vi "CNC Main.vi"() -> ()   [LabVIEW 2014]
uses:
  Typedefs/DXF Choices.ctl
  Typedefs/Demo States.ctl
  Typedefs/Motion Parameters.ctl
  <vilib>/Motion/Express/_s/nimc.fb.straightLineMove.blendMode.ctl
  Typedefs/GCode Choices.ctl
  Typedefs/GCode Scale Options.ctl
  Typedefs/DXF Scale Options.ctl
  Typedefs/Message.ctl
  Typedefs/Demo Actions.ctl
  GCode Parser/GCode Command Cluster.ctl
  <vilib>/Motion/Express/_s/nimc.ex.read.readTrajectoryData.coordinate.vi
  <vilib>/Motion/Express/_s/nimc.ex.read.readTrajectoryData.axis.vi
  <vilib>/Motion/Express/_s/nimc.ex.straightLineMove.startStraightLineMove.coordinate.modeRelative.0.vi
  <vilib>/Motion/Express/_s/nimc.ex.resetPosition.resetPosition.coordinate.vi
  <vilib>/Motion/Express/_s/nimc.ex.straightLineMove.startStraightLineMove.coordinate.modeAbsolute.0.vi
  <vilib>/Motion/Express/_s/nimc.ex.read.readExecutionData.coordinate.vi
  <vilib>/Motion/Express/_s/nimc.ex.stopMove.stop.coordinate.modeDecelerate.vi
  <vilib>/Motion/BlockNode/FB.NIMotion.xnode
  Functional_Global/Typedef_FPGA_Interface_Action.ctl
  <vilib>/ptbypt/NI_PtbyPt.lvlib
panel:
  in  "GCode Choices":T1=enum."Statue"
  in  "DXF Choices 2":enum16{"NI Logo", "Mermaid", "Hummingbird"}(ring)
  in  "DXF Debug":T2={"Pos Scale"=30.0, "X Offset"=-350.0, "Y Offset"=-350.0}
  in  "GCODE Debug":T3={"Pos Scale"=8.0, "Vel Scale"=8.0, "G0 Velocity"=800.0, "X Offset"=0.0, "Y Offset"=0.0, "Z Offset"=0.0}
  in  "OK Button":bool
  in  "OK Button 2":bool
  in  "OK Button 3":bool
  in  "OK Button 4":bool
  in  "OK Button 5":bool
  in  "OK Button 6":bool
  in  "Pause":bool
  out "Axis Positions":T4(graph)
  in  "Disable Graph Update":bool
  in  "Clear XY Graph":bool
  out "# in queue":i32
  out "pos.[] out":dbl[](array[numeric]) format="%#.2f"
  out "Demo States":T5
  in  "Global Stop":bool=TRUE
  out "GCODE":i32(listbox)=-1
  in  "Tab":enum32{"DXF", "GCODE", "Setup", "Debug"}(tab)
  in  "DXF Scale Options":T2[](array[typedef])=[{"Pos Scale"=250.0, "X Offset"=-1025.0, "Y Offset"=-1500.0}, {"Pos Scale"=75.0, "X Offset"=-180.0, "Y Offset"=-300.0}, {"Pos Scale"=30.0, "X Offset"=-350.0, "Y Offset"=-350.0}]
  in  "DXF Options":T6={"Pen Up Z"=50.0, "Pen Down Z"=-10.0, "Speed"=1500.0, "Z Move Speed"=300.0}
  in  "Start DXF":bool
  in  "DXF Choices":T7 items=["NI Logo", "Mermaid", "Hummingbird", ""]
  in  "GCODE Scale Options":T3[](array[typedef])=[{"Pos Scale"=20.0, "Vel Scale"=20.0, "G0 Velocity"=800.0, "X Offset"=0.0, "Y Offset"=0.0, "Z Offset"=0.0}, {"Pos Scale"=2.0, "Vel Scale"=1.0, "G0 Velocity"=800.0, "X Offset"=-225.0, "Y Offset"=-225.0, "Z Offset"=0.0}, {"Pos Scale"=7.0, "Vel Scale"=7.0, "G0 Velocity"=800.0, "X Offset"=0.0, "Y Offset"=0.0, "Z Offset"=0.0}]
  in  "Start GCode":bool
  in  "GCODE Choices":T7 items=["Letter S", "Scorpion", "Statue", "", ""]
  in  "Set Home Point":bool
  in  "Reset Position":bool
  out "Error":errorcluster
  in  "Update Rate (ms)":u32=20
  in  "Buffer size":i32=2000
  in  "Cell Font:Size":u32=24
  in  "Display Row":i32=6
  out "stored home position":dbl[](array[numeric])
  in  "Quit":bool
  in  "Reset to":dbl[](array[numeric])=[0.0, 0.0, 0.0, 0.0]
  in  "Axis Resources":refnum<k21>[](array[refnum])=["Axis 1", "Axis 2", "Axis 3", "Axis 4"]
  out "Request Parameters":T8={"timeout"=-1.0, "acceleration"=8000.0, "deceleration"=8000.0, "accel. jerk"=80000.0, "decel. jerk"=80000.0, "blend mode"=10551334, "blend delay"=-1.0, "smoothing"=0.5, "last blend"=FALSE} {"blend mode" items=["At Profile Complete"=10551335, "At Deceleration"=10551334, "After Delay"=10551336]}
  in  "Acc Multiplier":dbl=10.0 format="%#_13g"
  in  "Jerk Multiplier":dbl=100.0 format="%#_13g"
  in  "Coordinate Space":refnum<k21>="Coordinate Space 1"
  out "F":dbl=800.0
  in  "Move (debug)":bool
  in  "debug velocity":dbl=750.0
  in  "debug pos":dbl[](array[numeric])=[0.0, 0.0, -200.0, 0.0]
  in  "VEL %":dbl(slide)=1.0 min=0.01 max=1000.0 scale=0.01..100.0
  in  "Find Home":bool
  out "XY Graph":cluster{"X Array":dbl[], "Y Array":dbl[]}(graph)
  in  "Stop":bool
  out "Axis Velocities":T10(graph)
  # "scorpion:\n\nPOs: 2.5\nVel: 1\n\nAcc/Dec: 50000\nJerk: 500000\n\nG0: 800"
  # "X"
  # "Y"
  # "Z"
  # "Status:"
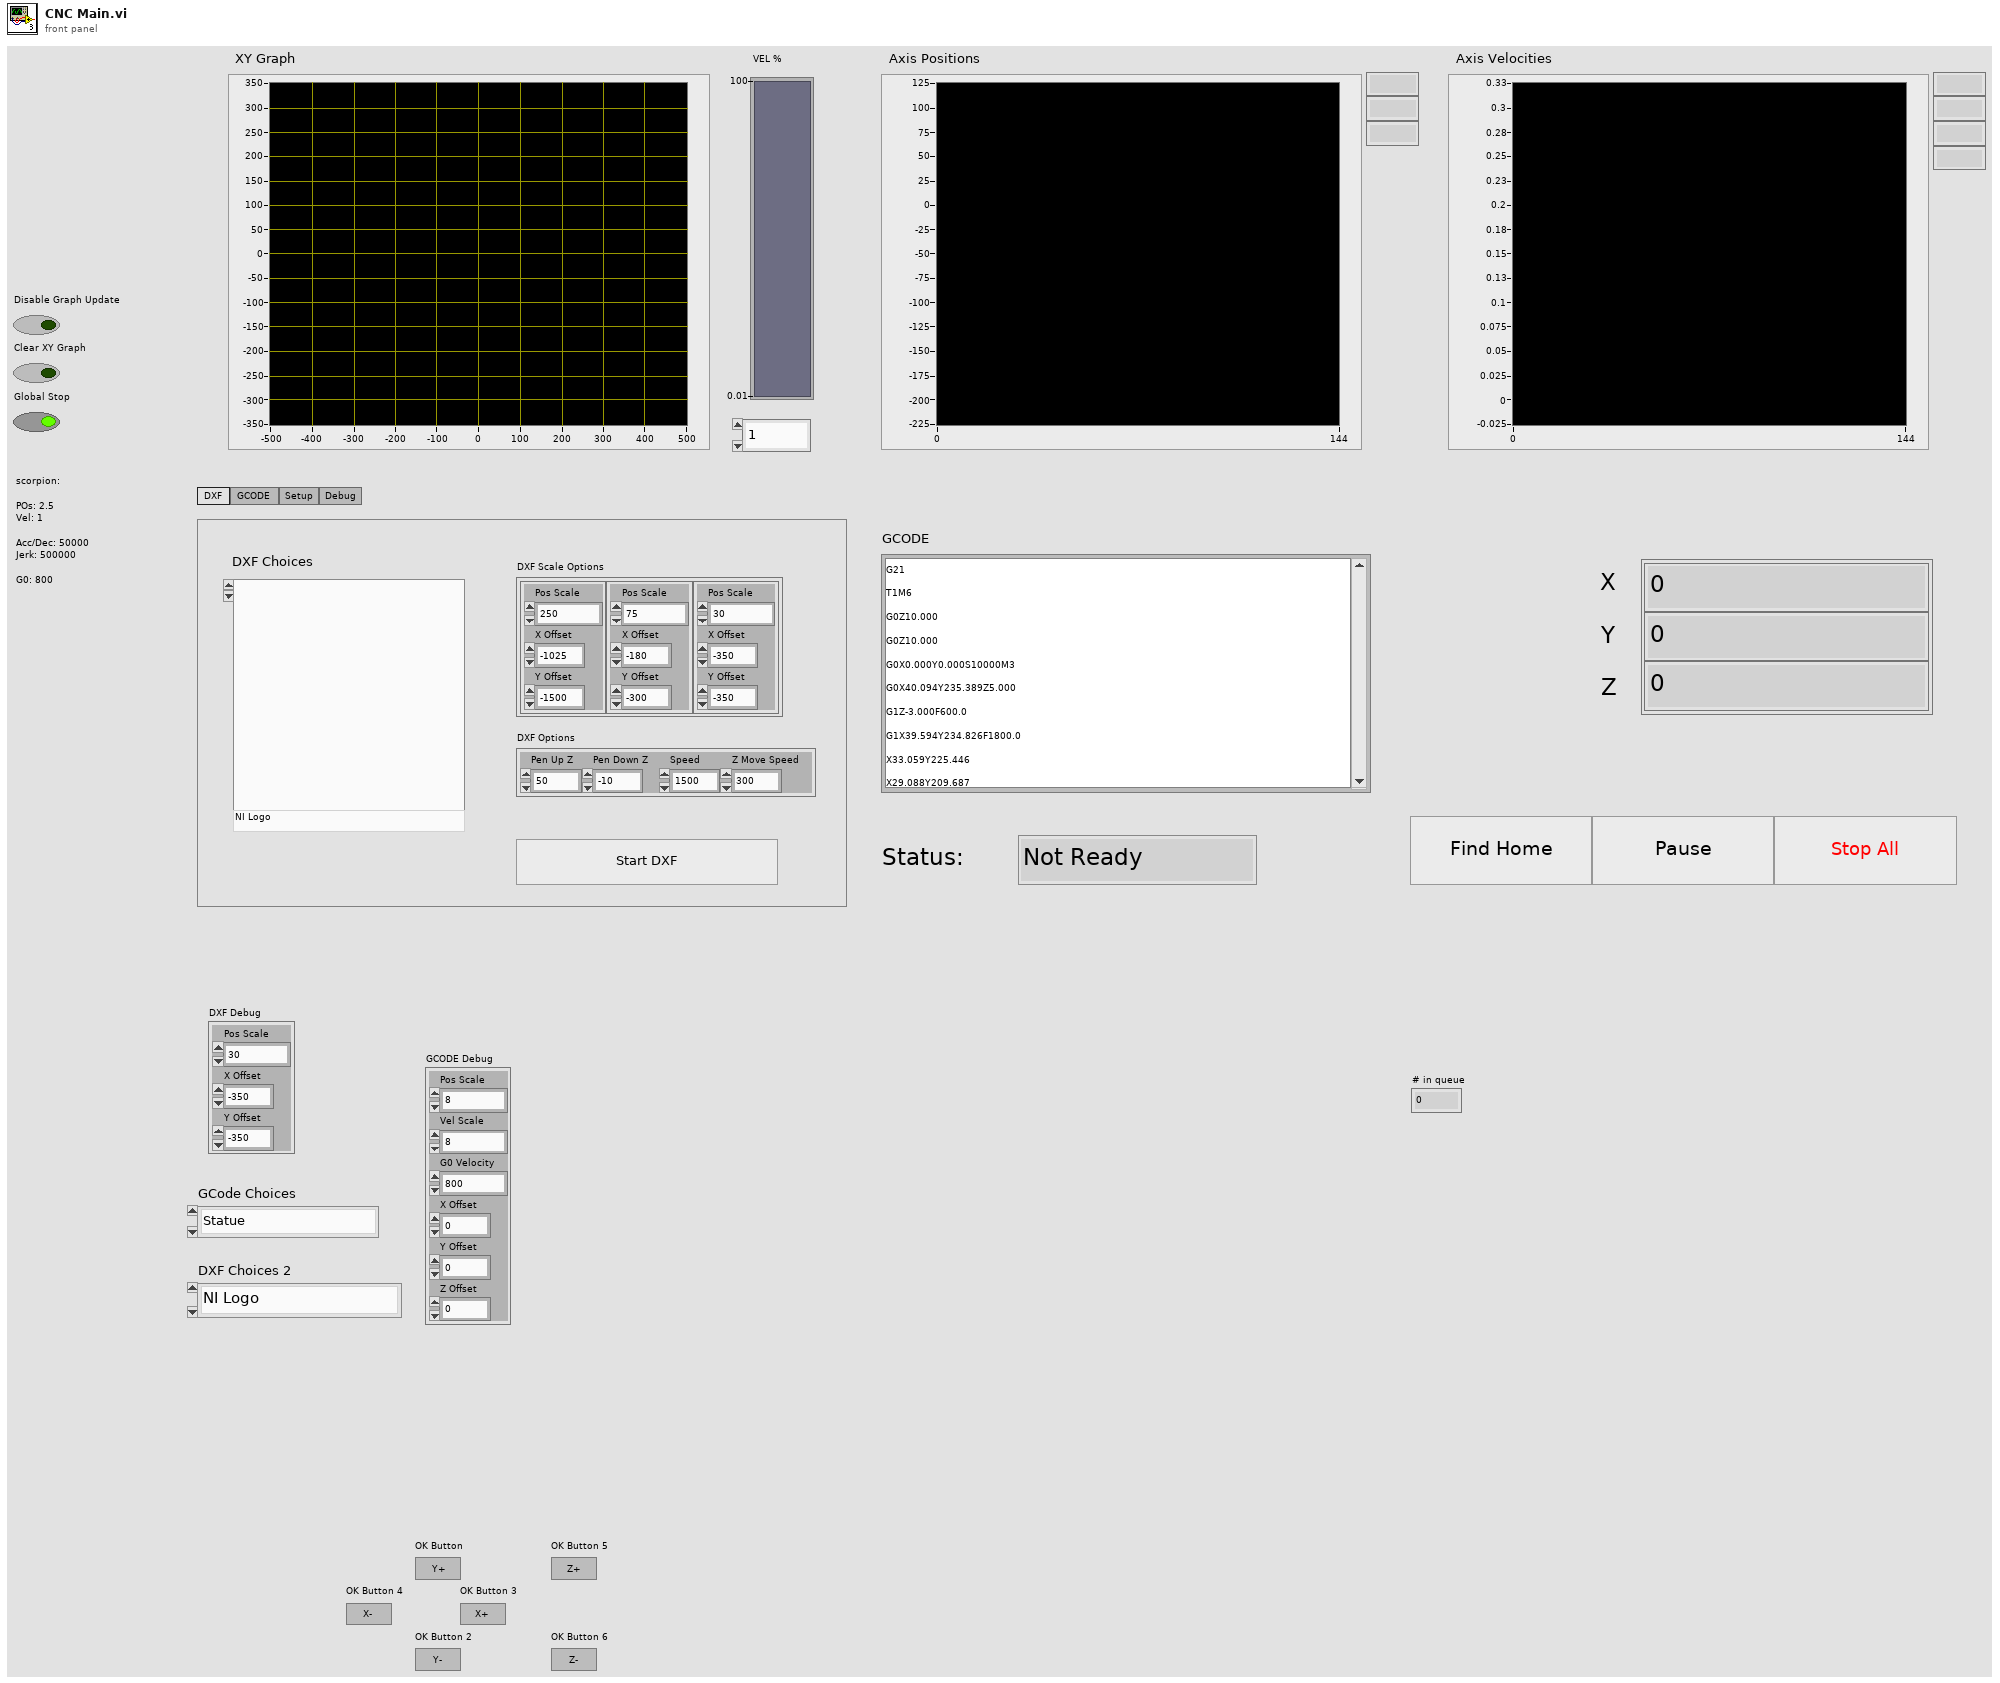
[diagram p1: front panel]
types:
  T1 = typedef "GCode Choices.ctl" = enum16{"S", "Scorpion", "Statue"}
  T2 = typedef "DXF Scale Options.ctl" = cluster{"Pos Scale":dbl, "X Offset":dbl, "Y Offset":dbl}
  T3 = typedef "GCode Scale Options.ctl" = cluster{"Pos Scale":dbl, "Vel Scale":dbl, "G0 Velocity":dbl, "X Offset":dbl, "Y Offset":dbl, "Z Offset":dbl}
  T4 = cluster{"commanded pos.[] out[0]":dbl, "commanded pos.[] out[1]":dbl, "commanded pos.[] out[2]":dbl}
  T5 = typedef "Demo States.ctl" = enum16{"Not Ready", "Ready (Idle)", "Running", "Paused"}
  T6 = cluster{"Pen Up Z":dbl, "Pen Down Z":dbl, "Speed":dbl, "Z Move Speed":dbl}
  T7 = typedef "DXF Choices.ctl" = u16
  T8 = typedef "Motion Parameters.ctl" = cluster{"timeout":dbl, "acceleration":dbl, "deceleration":dbl, "accel. jerk":dbl, "decel. jerk":dbl, "blend mode":T9, "blend delay":dbl, "smoothing":dbl, "last blend":bool}
  T9 = typedef "nimc.fb.straightLineMove.blendMode.ctl" = i32
  T10 = cluster{"[0]":dbl, "[1]":dbl, "[2]":dbl, "[3]":dbl}
  T11 = typedef "GCode Command Cluster.ctl" = cluster{"N":dbl, "GCODE":string, "X":dbl, "Y":dbl, "Z":dbl, "E":dbl, "I":dbl, "J":dbl, "S":dbl, "F":dbl, "Text":string, "G0 Vel":dbl}
  T12 = typedef "Message.ctl" = cluster{"Demo Actions":T13, "Data":variant}
  T13 = typedef "Demo Actions.ctl" = enum16{"Default (Null)", "Move (debug)", "Reset Position", "Find Home and Move to Zero", "Set Home Point", "Start", "Stop", "Pause", "Unpause"}
  T14 = typedef "Typedef_FPGA_Interface_Action.ctl" = enum16{"Initialize FPGA", "Get FPGA Reference", "Close FPGA"}
  T15 = enum8{"Enabled", "Disabled", "Disabled and Grayed Out"}
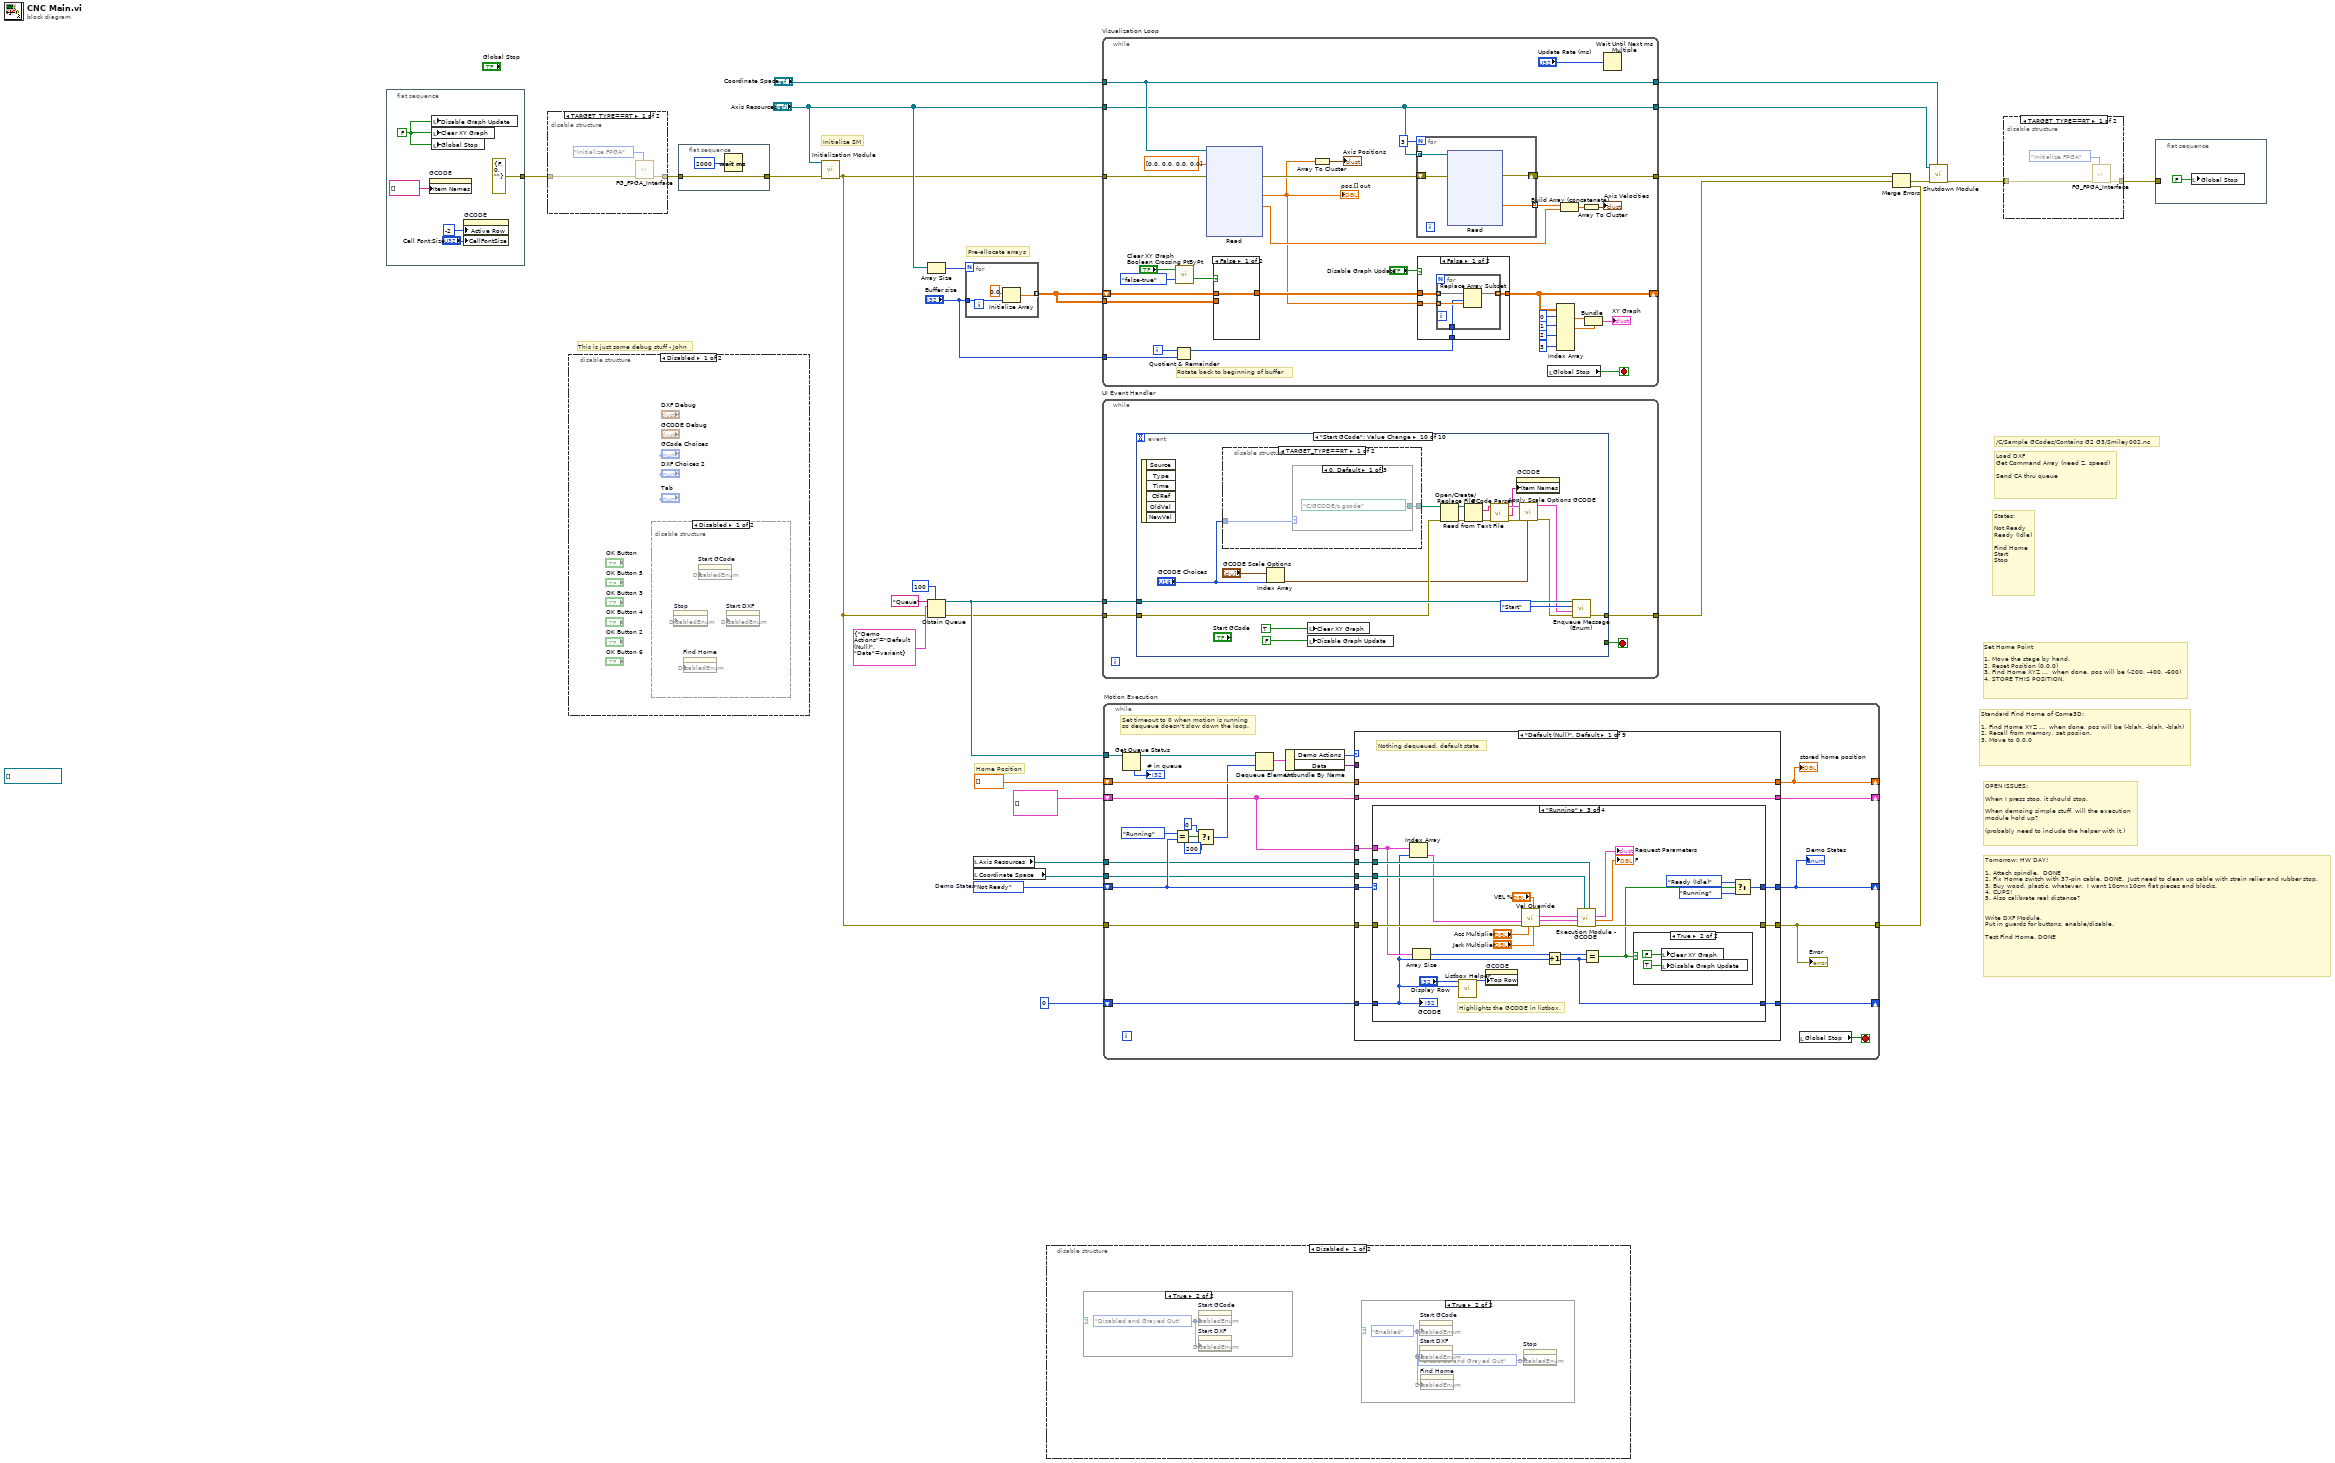
[diagram p0: block diagram]
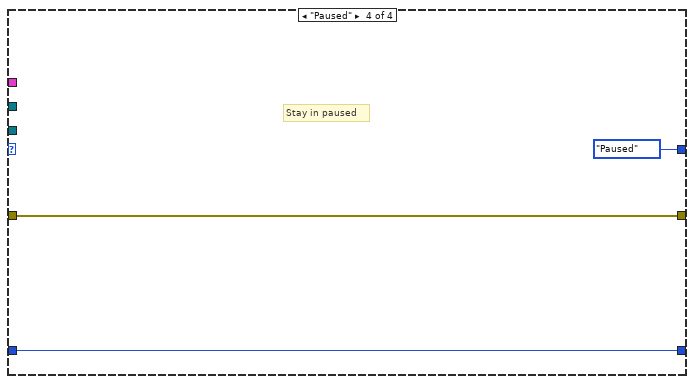
[diagram p12: hidden frame]
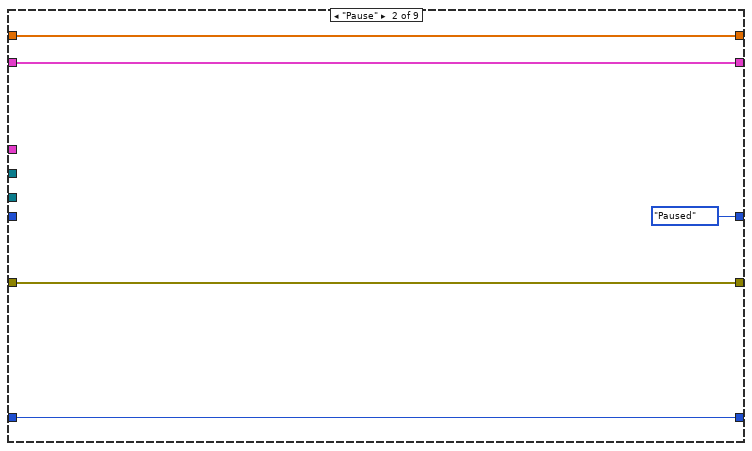
[diagram p13: hidden frame]
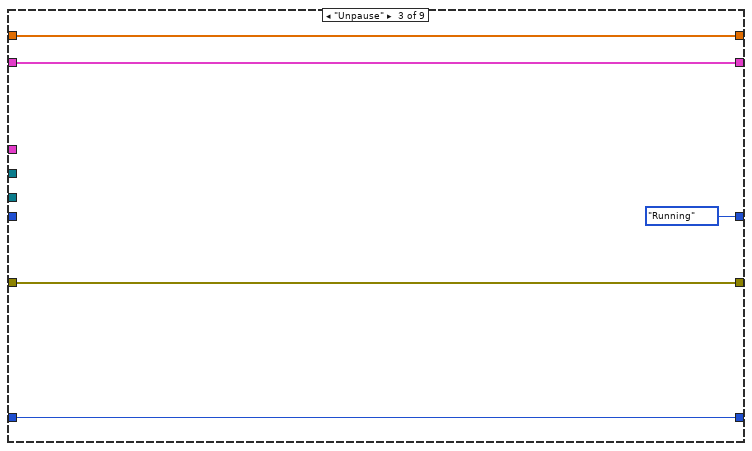
[diagram p14: hidden frame]
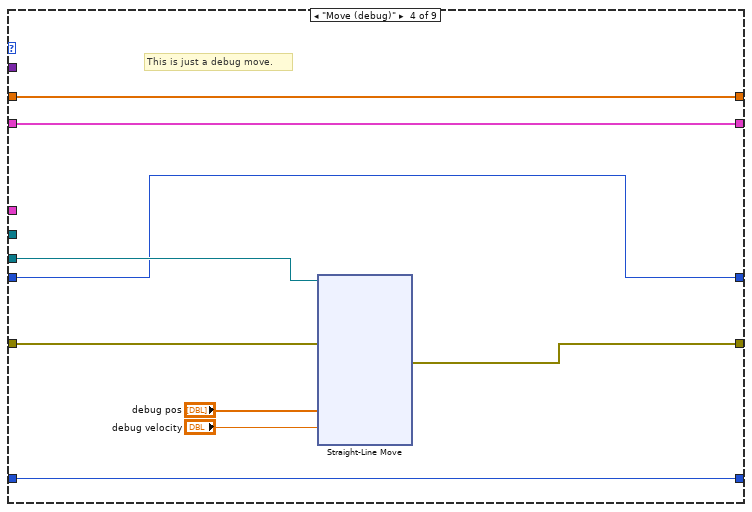
[diagram p15: hidden frame]
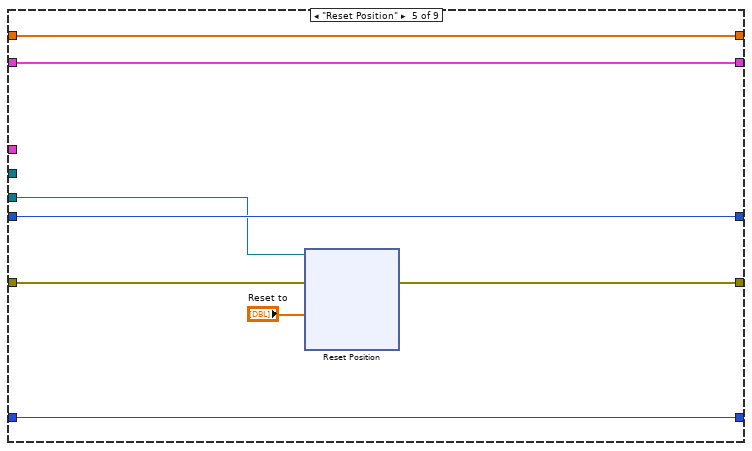
[diagram p16: hidden frame]
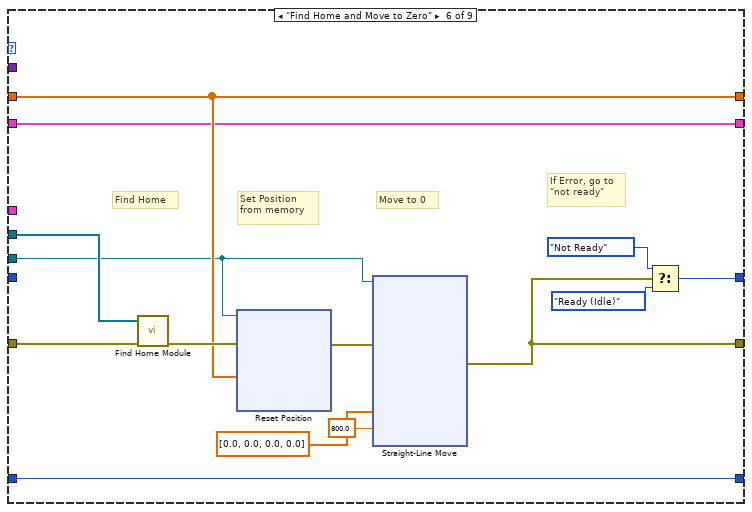
[diagram p17: hidden frame]
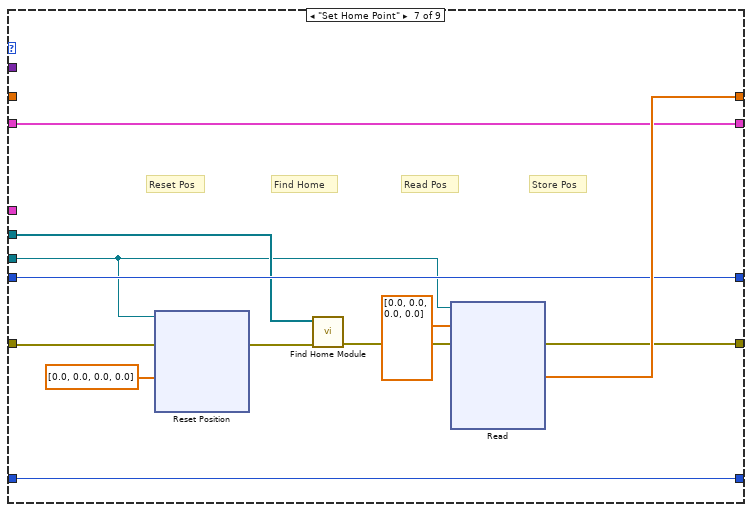
[diagram p18: hidden frame]
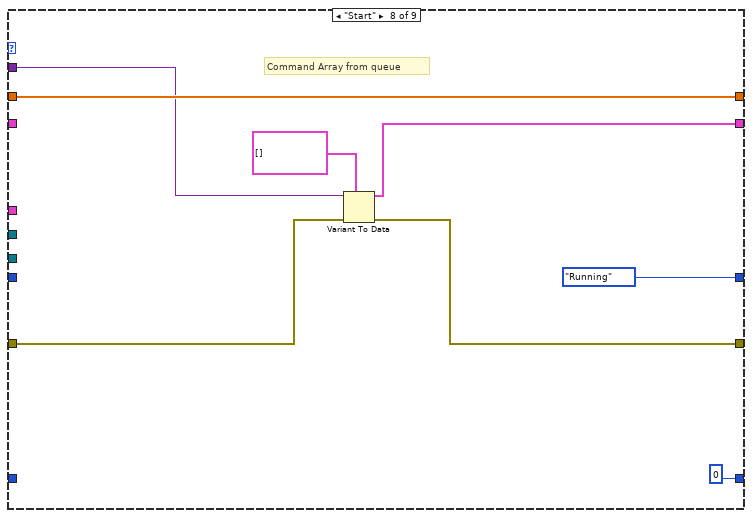
[diagram p19: hidden frame]
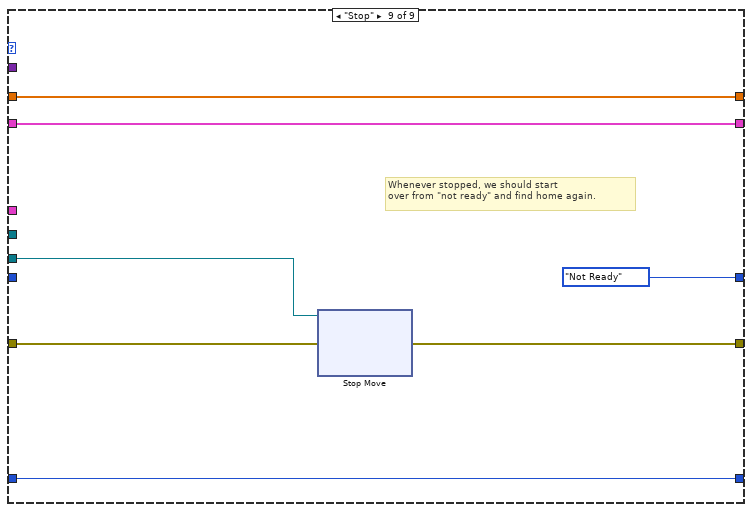
[diagram p20: hidden frame]
diagram:
  w4 = Demo_States."Not Ready"  # Demo States
  (unwired) refnum<k21>[] []
  # "This is just some debug stuff - John"
  # "Tomorrow: HW DAY!\n\n1. Attach spindle.  DONE\n2. Fix Home switch with 37-pin cable. DONE.  Just need to clean up cable with strain relier and rubber stop.\n3. Buy wood, plastic, whatever.  I want 10cmx10cm flat pieces and blocks.\n4. CLIPS!\n5. Also calibrate real distance?\n\n\nWrite DXF Module.\nPut in guards for buttons, enable/disable.\n\nTest Find Home. DONE"
  # "OPEN ISSUES:\n\nWhen I press stop, it should stop.\n\nWhen demoing simple stuff, will the execution \nmodule hold up?\n\n(probably need to include the helper with it.)"
  # "/C/Sample GCodes/Contains G2 G3/Smiley002.nc"
  # "Home Position"
  # "Pre-allocate arrays"
  # "Standard Find Home of Come3D:\n\n1. Find Home XYZ ...  when done, pos will be (-blah, -blah, -blah)\n2. Recall from memory, set posiion.\n3. Move to 0,0,0"
  # "Set Home Point\n\n1. Move the stage by hand.\n2. Reset Position (0,0,0)\n3. Find Home XYZ ...  when done, pos will be (-200, -400, -600)\n4. STORE THIS POSITION."
  # "Load DXF\nGet Command Array (need Z, speed)\n\nSend CA thru queue"
  # "States:\n\nNot Ready\nReady (Idle)\n\nFind Home\nStart\nStop"
  # "Initialize SM"
  n1 = flat-sequence {
    tunnel: [errorcluster {"status"=FALSE, "code"=0, "source"=""} ("error in")] -> w20
    frame #0 {
      w30 = FALSE ("Global Stop")
      n2 = property on="GCODE" class="LstBox (strict)"("Item Names"=string[] []) -> ()  [unwired: 2 in, 2 out]
      n3 = local write "Disable Graph Update"(w30) -> ()
      n4 = local write "Clear XY Graph"(w30) -> ()
      n5 = local write "Global Stop"(w30) -> ()
      n6 = property on="GCODE" class="LstBox (strict)"("Active Row"=-2 ("Active Row:Active Row Number"), "CellFontSize"="Cell Font:Size") -> ()  [unwired: 2 in, 2 out]
    }
  }
  n7 = disable-structure shown="TARGET_TYPE==RT" {
    disable-tunnel: [w35 w37] -> w28
    disable-tunnel: w20 -> [w34 w37]
    frame condition #0 {
      n8 = call "FG_FPGA_Interface.vi"("Action"=Typedef_FPGA_Interface_Action."Initialize FPGA", "error in"=w34) -> ("error out"=w35:errorcluster)  [unwired: 8 in, 1 out]
    }
    frame condition #1 (active) {
    }
  }
  n9 = disable-structure shown="Disabled" {
    frame Disabled {
      n10 = disable-structure shown="Disabled" {
        frame Disabled {
          n11 = property on="Stop" class="Bool" props=["DisabledEnum"]() -> ()  [unwired: 3 in, 2 out]
          n12 = property on="Find Home" class="Bool" props=["DisabledEnum"]() -> ()  [unwired: 3 in, 2 out]
          n13 = property on="Start GCode" class="Bool" props=["DisabledEnum"]() -> ()  [unwired: 3 in, 2 out]
          n14 = property on="Start DXF" class="Bool" props=["DisabledEnum"]() -> ()  [unwired: 3 in, 2 out]
        }
        frame Enabled {
        }
      }
    }
    frame Enabled {
    }
  }
  n15 = flat-sequence {
    tunnel: w28 -> [w38]
    tunnel: [w38] -> w25
    frame #0 {
      n16 = Wait (ms)(milliseconds to wait=u32 2000) -> ()  [unwired: 1 out]
    }
  }
  n17 = call "Initialization Module.vi"("error in (no error)"=w25, "Axis Resources In"="Axis Resources") -> ("error out"=w8:errorcluster)  [unwired: 8 in, 1 out]
  n18 = Array Size(array="Axis Resources") -> (size(s)=w27:i32)
  n19 = Obtain Queue(max queue size (-1, unlimited)=100, name (unnamed)="Queue", element data type=T12 {"Demo Actions"=enum."Default (Null)", "Data"=variant}, error in (no error)=w8) -> (queue out=w15:refnum<queue>, error out=w14:errorcluster)  [unwired: 1 in, 1 out]
  n20 = for {
    N: w27 -> [_]
    tunnel: [w41] -> w9 mode=indexing
    tunnel: "Buffer size" -> [w40]
    n21 = Initialize Array(0.0 ("element"), w40) -> (w41:dbl[])
  }
  n22 = local read "Axis Resources"() -> (w6:refnum<k21>[])
  n23 = local read "Coordinate Space"() -> (w5:refnum<k21>)
  n24 = disable-structure shown="Disabled" {
    frame Disabled {
      n25 = case shown="True" {
        selector: _ -> [_ _]
        frame False {
        }
        frame True {
          w43 = T15."Disabled and Grayed Out" ("Disabled")
          n26 = property on="Start GCode" class="Bool"("DisabledEnum"=w43) -> ()  [unwired: 2 in, 2 out]
          n27 = property on="Start DXF" class="Bool"("DisabledEnum"=w43) -> ()  [unwired: 2 in, 2 out]
        }
      }
      n28 = case shown="True" {
        selector: _ -> [_ _]
        frame False {
        }
        frame True {
          w45 = T15."Enabled" ("Disabled")
          n29 = property on="Start GCode" class="Bool"("DisabledEnum"=w45) -> ()  [unwired: 2 in, 2 out]
          n30 = property on="Start DXF" class="Bool"("DisabledEnum"=w45) -> ()  [unwired: 2 in, 2 out]
          n31 = property on="Find Home" class="Bool"("DisabledEnum"=w45) -> ()  [unwired: 2 in, 2 out]
          n32 = property on="Stop" class="Bool"("DisabledEnum"=T15."Disabled and Grayed Out" ("Disabled")) -> ()  [unwired: 2 in, 2 out]
        }
      }
    }
    frame Enabled {
    }
  }
  n33 = while "Visualization Loop" {
    tunnel: "Buffer size" -> [w78]
    tunnel: "Axis Resources" -> [w50]
    shift-right: [w59] -> _
    shift-left: w9 -> [w58]
    tunnel: "Coordinate Space" -> [w65]
    tunnel: [w50] -> w23
    tunnel: [w65] -> w24
    tunnel: w9 -> [w57]
    tunnel: w8 -> [w76]
    tunnel: [w74] -> w19
    i -> [w77]
    stop <- w62 stop-if-true
    # "Rotate back to beginning of buffer"
    n34 = Quotient & Remainder(x=w77, y=w78) -> (x-y*floor(x/y)=w73:i32)  [unwired: 1 out]
    n35 = call <vilib>:"Boolean Crossing PtByPt.vi"("direction"=enum16{"either", "false-true", "true-false"}."false-true", "input"="Clear XY Graph") -> ("crossing"=w54:bool)  [unwired: 1 in]
    n36 = xnode ("Read")("resource"=w65, "commanded pos.[]"=dbl[] [0.0, 0.0, 0.0, 0.0], "error in"=w76) -> ("commanded pos.[] out"=w46:dbl[], "commanded vel."=w49:dbl, "error out"=w75:errorcluster)  [unwired: 3 out]
    "pos.[] out" <- w46
    n37 = case shown="False" w54 {
      tunnel: w58 -> [w88 _]
      tunnel: w57 -> [_ w89]
      tunnel: [w88 w89] -> w56
      frame False {
      }
      frame True {
      }
    }
    n38 = Array To Cluster(array=w46) -> (cluster=→"Axis Positions":T4)
    n39 = for {
      N: 3 -> [_]
      tunnel: w50 -> [w102] mode=indexing
      tunnel: [w99] -> w61 mode=indexing
      shift-right: [w100] -> w74
      shift-left: w75 -> [w101]
      n40 = xnode ("Read")("resource"=w102, "error in"=w101) -> ("commanded vel."=w99:dbl, "error out"=w100:errorcluster)  [unwired: 3 out]
    }
    n41 = case shown="False" "Disable Graph Update" {
      tunnel: w73 -> [w82 _]
      tunnel: w46 -> [w81 _]
      tunnel: [w80 w87] -> w59
      tunnel: w56 -> [w79 w87]
      frame False {
        n42 = for {
          tunnel: w79 -> [w86] mode=indexing
          tunnel: w81 -> [w85] mode=indexing
          tunnel: w82 -> [w84]
          tunnel: [w83] -> w80 mode=indexing
          n43 = Replace Array Subset(array=w86, new element=w85, index=w84) -> (w83:dbl[])
        }
      }
      frame True {
      }
    }
    n44 = local read "Global Stop"() -> (w62:bool)
    n45 = Index Array(array=w59, index (row) #1=0 ("index (row)"), index (row) #2=1 ("index (row)"), index (row) #3=2 ("index (row)"), index (row) #4=3 ("index (row)")) -> (element #1=w68:dbl[], element #2=w69:dbl[])  [unwired: 4 in, 2 out]
    n46 = Build Array (concatenate)(w61, w49) -> (w60:dbl[])
    n47 = Array To Cluster(array=w60) -> (cluster=→"Axis Velocities":T10)
    n48 = Bundle(w68, w69) -> (→"XY Graph":cluster{dbl[], dbl[]})  [unwired: 1 in]
    n49 = Wait Until Next ms Multiple(millisecond multiple="Update Rate (ms)") -> ()  [unwired: 1 out]
  }
  n50 = while "UI Event Handler" {
    tunnel: w15 -> [w113]
    tunnel: w14 -> [w112]
    tunnel: [w111] -> w17
    stop <- w110 stop-if-true
    n51 = event shown="[9] \"Start GCode\": Value Change" {
      selector: _ -> [_ _ _ _ _ _ _ _ _ _]
      dyn-events: _ -> [_ _ _ _ _ _ _ _ _ _]
      timeout: _ -> [_ _ _ _ _ _ _ _ _ _]
      tunnel: w113 -> [_ w118 w122 w128 w135 w139 _ w146 w166 w203]
      tunnel: w112 -> [w114 w117 w121 w127 w134 w138 w142 w145 w162 w197]
      tunnel: [w114 w116 w120 w126 w133 w137 w142 w144 w165 w202] -> w111
      tunnel: [_ _ _ _ _ _ TRUE _ _ _] -> w110
      event Timeout {
        n52 = event-data() -> ()  [unwired: 1 in, 3 out]
      }
      event "Find Home": Value Change {
        n53 = event-data() -> ()  [unwired: 1 in, 6 out]
        n54 = call "Enqueue Message (Enum).vi"("error in (no error)"=w117, "Demo Actions"=Demo_Actions."Find Home and Move to Zero", "queue in"=w118) -> ("error out"=w116:errorcluster)  [unwired: 7 in, 1 out]
      }
      event "Set Home Point": Value Change {
        n55 = event-data() -> ()  [unwired: 1 in, 6 out]
        n56 = call "Enqueue Message (Enum).vi"("error in (no error)"=w121, "Demo Actions"=Demo_Actions."Set Home Point", "queue in"=w122) -> ("error out"=w120:errorcluster)  [unwired: 7 in, 1 out]
      }
      event "Stop": Value Change {
        n57 = event-data() -> ()  [unwired: 1 in, 6 out]
        n58 = call "Enqueue Message (Enum).vi"("error in (no error)"=w127, "Demo Actions"=Demo_Actions."Stop", "queue in"=w128) -> ("error out"=w126:errorcluster)  [unwired: 7 in, 1 out]
        n59 = local write "Clear XY Graph"(FALSE ("Clear XY Graph")) -> ()
        n60 = local write "Disable Graph Update"(TRUE ("No Update")) -> ()
      }
      event "Pause": Value Change {
        n61 = event-data() -> ()  [unwired: 1 in, 6 out]
        n62 = Select(t=Demo_Actions."Pause" ("Demo Actions"), s="Pause", f=Demo_Actions."Unpause" ("Demo Actions")) -> (s? t:f=w130:T13)
        n63 = call "Enqueue Message (Enum).vi"("error in (no error)"=w134, "Demo Actions"=w130, "queue in"=w135) -> ("error out"=w133:errorcluster)  [unwired: 7 in, 1 out]
      }
      event "Move (debug)": Value Change {
        n64 = event-data() -> ()  [unwired: 1 in, 6 out]
        n65 = call "Enqueue Message (Enum).vi"("error in (no error)"=w138, "Demo Actions"=Demo_Actions."Move (debug)", "queue in"=w139) -> ("error out"=w137:errorcluster)  [unwired: 7 in, 1 out]
      }
      event "Quit": Value Change {
        n66 = event-data() -> ()  [unwired: 1 in, 6 out]
        n67 = local write "Global Stop"(TRUE ("Global Stop")) -> ()
      }
      event "Reset Position": Value Change {
        n68 = event-data() -> ()  [unwired: 1 in, 6 out]
        n69 = call "Enqueue Message (Enum).vi"("error in (no error)"=w145, "Demo Actions"=Demo_Actions."Reset Position", "queue in"=w146) -> ("error out"=w144:errorcluster)  [unwired: 7 in, 1 out]
      }
      event "Start DXF": Value Change {
        n70 = event-data() -> ()  [unwired: 1 in, 6 out]
        n71 = disable-structure shown="TARGET_TYPE==Windows, Default" {
          disable-tunnel: [w168 w172] -> w150
          disable-tunnel: "DXF Choices" -> [w167 w174]
          frame condition #0 {
            n72 = case shown="0, Default" w167 {
              tunnel: [path "C:/DXF/NI.dxf" ("file path (use dialog)") path "C:/DXF/mermaid.dxf" ("file path (use dialog)") path "C:/DXF/hummingbird.dxf" ("file path (use dialog)")] -> w168
              frame 0, Default {
              }
              frame 1 {
              }
              frame 2 {
              }
            }
          }
          frame condition #1 (active) {
            n73 = call "Example files directory.vi"("File Type"=enum16{"DXF", "GCODE"}."DXF") -> ("path"=w173:path)  [unwired: 10 in]
            n74 = case shown="1" w174 {
              tunnel: w173 -> [w178 w181 w184]
              tunnel: [w176 w179 w182] -> w172
              frame 0, Default {
                n75 = Build Path(base path=w178, name or relative path="NI.dxf") -> (appended path=w176:path)
              }
              frame 1 {
                n76 = Build Path(base path=w181, name or relative path="mermaid.dxf") -> (appended path=w179:path)
              }
              frame 2 {
                n77 = Build Path(base path=w184, name or relative path="hummingbird.dxf") -> (appended path=w182:path)
              }
            }
          }
        }
        n78 = Index Array(array="DXF Scale Options", index="DXF Choices") -> (element=w148:T2)
        n79 = local write "Clear XY Graph"(TRUE ("Clear XY Graph")) -> ()
        n80 = local write "Disable Graph Update"(FALSE ("No Update")) -> ()
        n81 = Open/Create/Replace File(file path (use dialog)=w150, error in=w162) -> (refnum out=w164:refnum<file>, error out=w163:errorcluster)  [unwired: 4 in, 1 out]
        n82 = Read from Text File(file (use dialog)=w164, error in=w163) -> (text=w157:string, error out=w158:errorcluster)  [unwired: 2 in, 2 out]
        n83 = call "Load DXF 2.vi"("DXF Options"="DXF Options", "error in (no error)"=w158, "String in"=w157) -> ("error out"=w152:errorcluster, "String Array"=w156:string[], "Command Array"=w155:T11[])  [unwired: 6 in]
        n84 = call "Apply Scale Options DXF.vi"("Scale Options"=w148, "error in (no error)"=w152, "Command Array"=w155) -> ("error out"=w153:errorcluster, "Command Array Out"=w154:T11[])  [unwired: 7 in]
        n85 = property on="GCODE" class="LstBox (strict)"("Item Names"=w156) -> ()  [unwired: 2 in, 2 out]
        n86 = call "Enqueue Message (Enum).vi"("error in (no error)"=w153, "Message Data"=w154, "Demo Actions"=Demo_Actions."Start", "queue in"=w166) -> ("error out"=w165:errorcluster)  [unwired: 6 in, 1 out]
      }
      event "Start GCode": Value Change {
        n87 = event-data() -> ()  [unwired: 1 in, 6 out]
        n88 = disable-structure shown="TARGET_TYPE==RT" {
          disable-tunnel: [w205 w212] -> w188
          disable-tunnel: "GCODE Choices" -> [w204 w211]
          frame condition #0 {
            n89 = case shown="0, Default" w204 {
              tunnel: [path "C:/GCODE/s.gcode" ("file path (use dialog)") path "C:/GCODE/Scorpion.gcode" ("file path (use dialog)") path "C:/GCODE/statue.gcode" ("file path (use dialog)")] -> w205
              frame 0, Default {
              }
              frame 1 {
              }
              frame 2 {
              }
            }
          }
          frame condition #1 (active) {
            n90 = call "Example files directory.vi"("File Type"=enum16{"DXF", "GCODE"}."GCODE") -> ("path"=w209:path)  [unwired: 10 in]
            n91 = case shown="2" w211 {
              tunnel: [w213 w216 w219] -> w212
              tunnel: w209 -> [w214 w217 w220]
              frame 0, Default {
                n92 = Build Path(base path=w214, name or relative path="s.gcode") -> (appended path=w213:path)
              }
              frame 1 {
                n93 = Build Path(base path=w217, name or relative path="scorpion.gcode") -> (appended path=w216:path)
              }
              frame 2 {
                n94 = Build Path(base path=w220, name or relative path="statue.gcode") -> (appended path=w219:path)
              }
            }
          }
        }
        n95 = Index Array(array="GCODE Scale Options", index="GCODE Choices") -> (element=w186:T3)
        n96 = local write "Clear XY Graph"(TRUE ("Clear XY Graph")) -> ()
        n97 = local write "Disable Graph Update"(FALSE ("No Update")) -> ()
        n98 = Open/Create/Replace File(file path (use dialog)=w188, error in=w197) -> (refnum out=w201:refnum<file>, error out=w198:errorcluster)  [unwired: 4 in, 1 out]
        n99 = Read from Text File(file (use dialog)=w201, error in=w198) -> (text=w200:string, error out=w199:errorcluster)  [unwired: 2 in, 2 out]
        n100 = call "GCode Parser.vi"("error in (no error)"=w199, "String in"=w200) -> ("error out"=w193:errorcluster, "String Array"=w191:string[], "Command Array"=w192:T11[])  [unwired: 7 in]
        n101 = property on="GCODE" class="LstBox (strict)"("Item Names"=w191) -> ()  [unwired: 2 in, 2 out]
        n102 = call "Apply Scale Options GCODE.vi"("Scale Options"=w186, "error in (no error)"=w193, "Command Array"=w192) -> ("error out"=w190:errorcluster, "Command Array Out"=w189:T11[])  [unwired: 7 in]
        n103 = call "Enqueue Message (Enum).vi"("error in (no error)"=w190, "Message Data"=w189, "Demo Actions"=Demo_Actions."Start", "queue in"=w203) -> ("error out"=w202:errorcluster)  [unwired: 6 in, 1 out]
      }
    }
  }
  n104 = while "Motion Execution" {
    tunnel: w15 -> [w239]
    shift-right: [w245] -> _
    shift-left: w4 -> [w232]
    shift-right: [w242] -> _
    shift-left: dbl[] [] ("position[] out") -> [w241]
    shift-right: [w235] -> _
    shift-left: T11[] [] ("Command Array") -> [w222]
    shift-right: [w234] -> _
    shift-left: 0 -> [w233]
    tunnel: w6 -> [w224]
    tunnel: w5 -> [w223]
    tunnel: w8 -> [w244]
    tunnel: [w243] -> w7
    stop <- w240 stop-if-true
    # "Set timeout to 0 when motion is running\nso dequeue doesn't slow down the loop."
    n105 = Get Queue Status(queue=w239) -> (queue out=w226:refnum<queue>, # elements in queue=→"# in queue":i32)  [unwired: 2 in, 6 out]
    n106 = Equal?(x=Demo_States."Running", y=w232) -> (x = y?=w229:bool)
    n107 = Select(t=0, s=w229, f=200) -> (s? t:f=w227:i32)
    n108 = Dequeue Element(queue=w226, timeout in ms (-1)=w227) -> (element=w238:T12)  [unwired: 1 in, 3 out]
    n109 = Unbundle By Name(w238) -> ("Demo Actions"=w237:T13, "Data"=w236:variant)
    n110 = case shown="\"Default (Null)\", Default" w237 {
      tunnel: w232 -> [w246 _ _ w304 w332 _ w383 _ _]
      tunnel: [w253 Demo_States."Paused" Demo_States."Running" w304 w332 w350 w383 Demo_States."Running" Demo_States."Not Ready"] -> w245
      tunnel: w244 -> [w255 w295 w300 w308 w331 w347 w380 w403 w413]
      tunnel: [w254 w295 w300 w307 w330 w346 w379 w402 w412] -> w243
      tunnel: [w256 w294 w299 w309 w329 w345 w385 w406 w411] -> w242
      tunnel: w241 -> [w256 w294 w299 w309 w329 w345 _ w406 w411]
      tunnel: w223 -> [w252 _ _ w305 w328 w340 w374 _ w410]
      tunnel: w236 -> [_ _ _ _ _ _ _ w405 _]
      tunnel: [w250 w293 w298 w303 w326 w342 w376 w404 w409] -> w235
      tunnel: w222 -> [w250 w293 w298 w303 w326 w342 w376 _ w409]
      tunnel: w224 -> [w251 _ _ _ _ w343 w378 _ _]
      tunnel: [w248 w292 w297 w302 w325 w341 w375 0 w408] -> w234
      tunnel: w233 -> [w249 w292 w297 w302 w325 w341 w375 _ w408]
      tunnel: w222 -> [w247 _ _ _ _ _ _ _ _]
      frame "Default (Null)", Default {
        # "Nothing dequeued, default state"
        n111 = case shown="\"Running\"" w246 {
          selector: w246 -> [w257 w260 _ _]
          tunnel: w255 -> [w259 w262 w280 w290]
          tunnel: [w259 w262 w285 w290] -> w254
          tunnel: [w257 w260 w284 Demo_States."Paused"] -> w253
          tunnel: w252 -> [_ _ w278 _]
          tunnel: w251 -> [_ _ w277 _]
          tunnel: w247 -> [_ _ w275 _]
          tunnel: w249 -> [w258 w261 w263 w289]
          tunnel: [w258 w261 w271 w289] -> w248
          frame "Not Ready", Default {
          }
          frame "Ready (Idle)" {
          }
          frame "Running" {
            # "Highlights the GCODE in listbox."
            n112 = Index Array(array=w275, index=w263) -> (element=w269:T11)
            n113 = Array Size(array=w275) -> (size(s)=w274:i32)
            n114 = call "Listbox Helper.vi"("Count In"=w263, "Display Row"="Display Row") -> ("Out"=w272:i32)  [unwired: 9 in]
            n115 = property on="GCODE" class="LstBox (strict)"("Top Row"=w272) -> ()  [unwired: 2 in, 2 out]
            n116 = call "Vel Override.vi"("Jerk Multiplier"="Jerk Multiplier", "VEL ADJ"="VEL %", "Acc Multiplier"="Acc Multiplier", "error in (no error)"=w280, "CMD In"=w269) -> ("error out"=w281:errorcluster, "CMD Out"=w267:T11, "output cluster"=w279:T8)  [unwired: 4 in]
            n117 = Increment(x=w263) -> (x+1=w271:i32)
            n118 = call "Execution Module - GCODE.vi"("Axis Resources"=w277, "Coordinate Space Resource"=w278, "error in (no error)"=w281, "GCode CMD"=w267, "Motion Parameters"=w279) -> ("error out"=w285:errorcluster, "Speed Request"=→"F":dbl, "Motion Parameters Out"=→"Request Parameters":T8)  [unwired: 4 in]
            n119 = Equal?(x=w274, y=w271) -> (x = y?=w270:bool)
            n120 = case shown="True" w270 {
              frame False {
              }
              frame True {
                n121 = local write "Clear XY Graph"(FALSE ("Clear XY Graph")) -> ()
                n122 = local write "Disable Graph Update"(TRUE ("No Update")) -> ()
              }
            }
            n123 = Select(t=Demo_States."Ready (Idle)", s=w270, f=Demo_States."Running") -> (s? t:f=w284:T5)
            "GCODE" <- w263
          }
          frame "Paused" {
            # "Stay in paused"
          }
        }
      }
      frame "Pause" {
      }
      frame "Unpause" {
      }
      frame "Move (debug)" {
        # "This is just a debug move."
        n124 = xnode ("Straight-Line Move")("position[]"="debug pos", "velocity"="debug velocity", "resource"=w305, "error in"=w308) -> ("error out"=w307:errorcluster)  [unwired: 6 in, 2 out]
      }
      frame "Reset Position" {
        n125 = xnode ("Reset Position")("position[]"="Reset to", "resource"=w328, "error in"=w331) -> ("error out"=w330:errorcluster)  [unwired: 2 out]
      }
      frame "Find Home and Move to Zero" {
        # "If Error, go to\n\"not ready\""
        # "Move to 0"
        # "Set Position\nfrom memory"
        # "Find Home"
        n126 = call "Find Home Module"("error in (no error)"=w347, "Array"=w343) -> ("error out"=w349:errorcluster)  [unwired: 9 in]
        n127 = xnode ("Reset Position")("position[]"=w345, "resource"=w340, "error in"=w349) -> ("error out"=w348:errorcluster)  [unwired: 2 out]
        n128 = xnode ("Straight-Line Move")("position[]"=dbl[] [0.0, 0.0, 0.0, 0.0], "velocity"=800.0, "resource"=w340, "error in"=w348) -> ("error out"=w346:errorcluster)  [unwired: 6 in, 2 out]
        n129 = Select(t=Demo_States."Not Ready", s=w346, f=Demo_States."Ready (Idle)") -> (s? t:f=w350:T5)
      }
      frame "Set Home Point" {
        # "Store Pos"
        # "Read Pos"
        # "Find Home"
        # "Reset Pos"
        n130 = xnode ("Reset Position")("position[]"=dbl[] [0.0, 0.0, 0.0, 0.0], "resource"=w374, "error in"=w380) -> ("error out"=w382:errorcluster)  [unwired: 2 out]
        n131 = call "Find Home Module"("error in (no error)"=w382, "Array"=w378) -> ("error out"=w381:errorcluster)  [unwired: 9 in]
        n132 = xnode ("Read")("resource"=w374, "position[]"=dbl[] [0.0, 0.0, 0.0, 0.0], "error in"=w381) -> ("position[] out"=w385:dbl[], "error out"=w379:errorcluster)  [unwired: 3 out]
      }
      frame "Start" {
        # "Command Array from queue"
        n133 = Variant To Data(error in=w403, type=T11[] [] ("Command Array"), Variant=w405) -> (data=w404:T11[], error out=w402:errorcluster)
      }
      frame "Stop" {
        # "Whenever stopped, we should start\nover from \"not ready\" and find home again."
        n134 = xnode ("Stop Move")("resource"=w410, "error in"=w413) -> ("error out"=w412:errorcluster)  [unwired: 1 in, 2 out]
      }
    }
    "Error" <- w243
    "Demo States" <- w245
    "stored home position" <- w242
    n135 = local read "Global Stop"() -> (w240:bool)
  }
  n136 = Merge Errors(w19, w17, w7) -> (w18:errorcluster)
  n137 = call "Shutdown Module.vi"("Coordinate Space"=w24, "error in (no error)"=w18, "Axis Resources In"=w23) -> ("error out"=w2:errorcluster)  [unwired: 7 in, 1 out]
  n138 = disable-structure shown="TARGET_TYPE==RT" {
    disable-tunnel: [w424 w426] -> w1
    disable-tunnel: w2 -> [w423 w426]
    frame condition #0 {
      n139 = call "FG_FPGA_Interface.vi"("Action"=Typedef_FPGA_Interface_Action."Initialize FPGA", "error in"=w423) -> ("error out"=w424:errorcluster)  [unwired: 8 in, 1 out]
    }
    frame condition #1 (active) {
    }
  }
  n140 = flat-sequence {
    tunnel: w1 -> [_]
    frame #0 {
      n141 = local write "Global Stop"(FALSE ("Global Stop")) -> ()
    }
  }
